vi "Test SenseHat Display Image.vi"() -> ()   [LabVIEW 2020]
uses:
  <vilib>/MakerHub/LINX/LMH-LINX.lvlib
  src/RPI.SenseHat.Display/Classes/SenseHat.Display/RPI.SenseHat.Display.lvclass
  src/RPI.SenseHat.Display/Classes/Image/Image.lvclass
  src/RPI.SenseHat.Display/Classes/Pixel/Pixel.lvclass
  src/RPI.SenseHat.Display/Classes/Color/Color.lvclass
  <vilib>/MakerHub/LINX/Public/Utilities/Open Local.vi
  src/RPI.SenseHat.Display/TypeDefs/Display Direction.ctl
  src/RPI.SenseHat.Display/RPI.SenseHat.Display.lvlib
panel:
  in  "Direction":T1
  in  "offset y":i32
  in  "offset x":i32
  in  "Array":u32[][](array[colorbox])
  out "Device Name":string
  out "Error Out":errorcluster
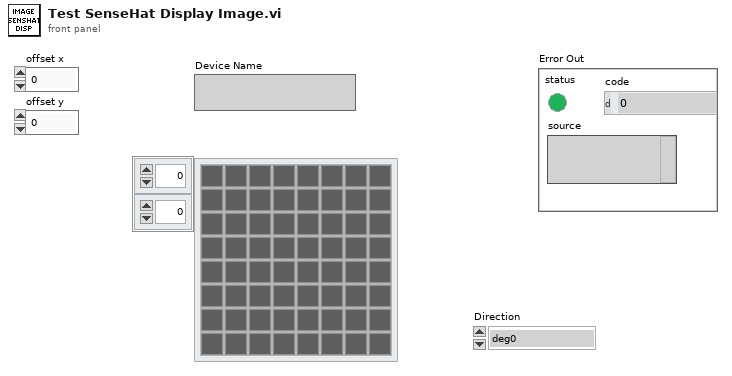
[diagram p1: front panel]
types:
  T1 = typedef "RPI.SenseHat.Display.lvlib/Display Direction.ctl" = enum16{"deg0", "deg90", "deg180", "deg270"}
  T2 = typedef "LMH-LINX.lvlib/LINX Ref.ctl" = cluster{"IO":T3, "Interface":T4, "LINX Device Config":T5}
  T3 = typedef "LMH-LINX.lvlib/Platform.ctl" = enum16{"Remote", "Local"}
  T4 = typedef "LMH-LINX.lvlib/Interface.ctl" = enum16{"Serial", "TCP"}
  T5 = typedef "LMH-LINX.lvlib/Device.lvlib/LINX Device Config.ctl" = cluster{"Interface":T4, "COM Port":refnum<visa-resource-name>, "TCP Configuration":T6, "Device Family":u8, "Device ID":u8, "Device Name":string, "TCP Ref":refnum<k5>, "Channels":T7}
  T6 = typedef "LMH-LINX.lvlib/Device.lvlib/TCP Config.ctl" = cluster{"IP Address":string, "Port":u16}
  T7 = typedef "LMH-LINX.lvlib/Channels.ctl" = cluster{"DI":u8[], "DO":u8[], "AI":u8[], "AO":u8[], "PWM":u8[], "QE":u8[], "UART":u8[], "I2C 2":u8[], "SPI":u8[], "CAN":u8[], "Servo":u8[], "AI Ref (V)":dbl, "AI Resolution (Bits)":u8, "AO Ref (V)":dbl, "AO Resolution (Bits)":u8}
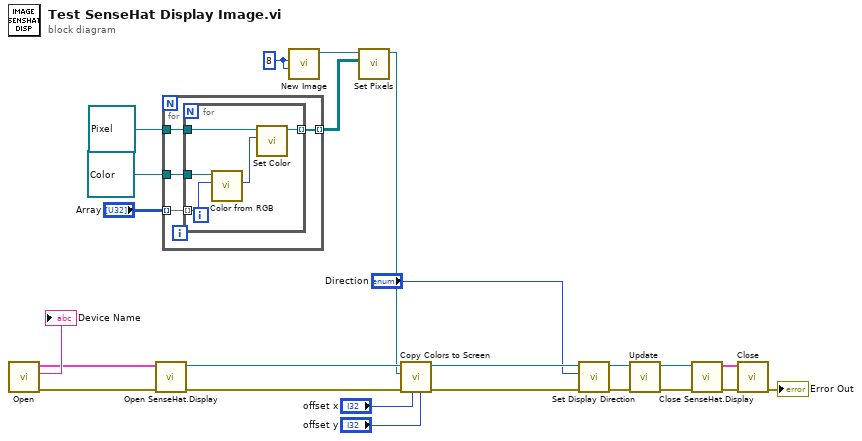
[diagram p0: block diagram]
diagram:
  w14 = 8 ("Height")
  n1 = call-poly <vilib>:"Open.vi"() -> ("Error Out"=w22:errorcluster, "Device Name"=→"Device Name":string, "LINX Resource"=w15:T2)  [unwired: 9 in]
  n2 = call "Open SenseHat.Display.vi"("error in (no error)"=w22, "LINX Resource"=w15) -> ("error out"=w21:errorcluster, "senseHatDisplay out"=w20:refnum<class "RPI.SenseHat.Display.lvclass">)  [unwired: 8 in]
  n3 = for {
    tunnel: "Array" -> [w28] mode=indexing
    tunnel: refnum<class "Color.lvclass"> refnum ("RPI.SenseHat.Display.lvlib:Color") -> [w27]
    tunnel: refnum<class "Pixel.lvclass"> refnum ("RPI.SenseHat.Display.lvlib:Pixel.lvclass") -> [w26]
    tunnel: [w25] -> w9 mode=indexing
    n4 = for {
      tunnel: w28 -> [w33] mode=indexing
      tunnel: w27 -> [w32]
      tunnel: w26 -> [w31]
      tunnel: [w29] -> w25 mode=indexing
      n5 = call "Color from RGB.vi"("Color Box"=w33, "Color in"=w32) -> ("Color"=w30:u16)  [unwired: 7 in, 2 out]
      n6 = call-dynamic "Set Color.vi"("Color"=w30, "Pixel in"=w31) -> ("Pixel out"=w29:refnum<class "Pixel.lvclass">)  [unwired: 8 in, 1 out]
    }
  }
  n7 = call "New Image.vi"("Height"=w14, "Width"=w14) -> ("Image out"=w13:refnum<class "Image.lvclass">)  [unwired: 8 in, 1 out]
  n8 = call "Set Pixels.vi"("Pixels"=w9, "Image in"=w13) -> ("Image out"=w8:refnum<class "Image.lvclass">)  [unwired: 8 in, 1 out]
  n9 = call "Copy Colors to Screen.vi"("offset y"="offset y", "offset x"="offset x", "error in (no error)"=w21, "Image"=w8, "senseHatDisplay in"=w20) -> ("error out"=w4:errorcluster, "senseHatDisplay out"=w5:refnum<class "RPI.SenseHat.Display.lvclass">)  [unwired: 5 in]
  n10 = call "Set Display Direction.vi"("error in (no error)"=w4, "Direction"="Direction", "senseHatDisplay in"=w5) -> ("error out"=w2:errorcluster, "senseHatDisplay out"=w3:refnum<class "RPI.SenseHat.Display.lvclass">)  [unwired: 7 in]
  n11 = call "Update.vi"("error in (no error)"=w2, "senseHatDisplay in"=w3) -> ("error out"=w18:errorcluster, "senseHatDisplay out"=w19:refnum<class "RPI.SenseHat.Display.lvclass">)  [unwired: 8 in]
  n12 = call "Close SenseHat.Display.vi"("error in (no error)"=w18, "senseHatDisplay in"=w19) -> ("error out"=w23:errorcluster, "LINX Resource"=w24:T2)  [unwired: 8 in]
  n13 = call <vilib>:"Close.vi"("Error In"=w23, "LINX Resource"=w24) -> ("Error Out"=→"Error Out":errorcluster)  [unwired: 9 in]
